vi "ExtWndAttributes.vi"(8 "EorIn":errorcluster) -> (0 "ErrOut":errorcluster)   [LabVIEW 2014]
doc: "Use this template to build a VI to use as a subVI."
panel:
  # "Output Parameters"
  # "Input Parameters"
  # "VI Description:\nThis VI is .."
  # ":: MVi Framework V1.0 ::\nAuthor:Gaoke Yang\nEmail: gaoke.yang@yahoo.com\nWeb: www.mvicontrol.com\nCopyright (C) 2015, MVI Technologies All Rights Reserved"
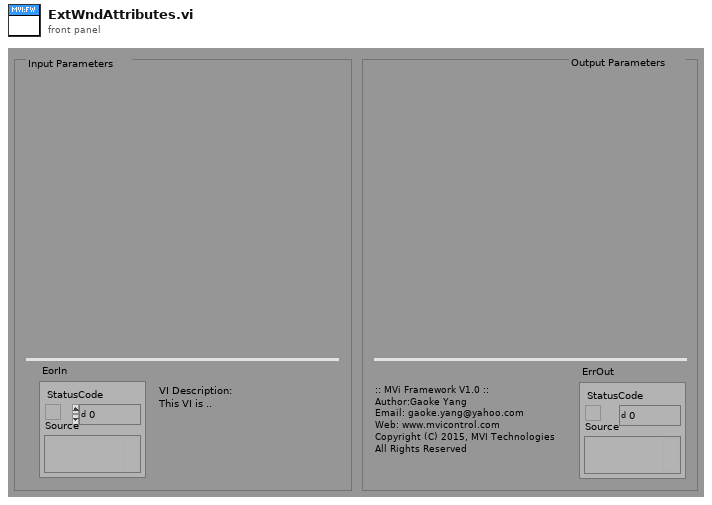
[diagram p1: front panel]
types:
  T1 = typedef "Image Type" = u32
  T2 = typedef "IMAQ Image.ctl" = refnum<image>
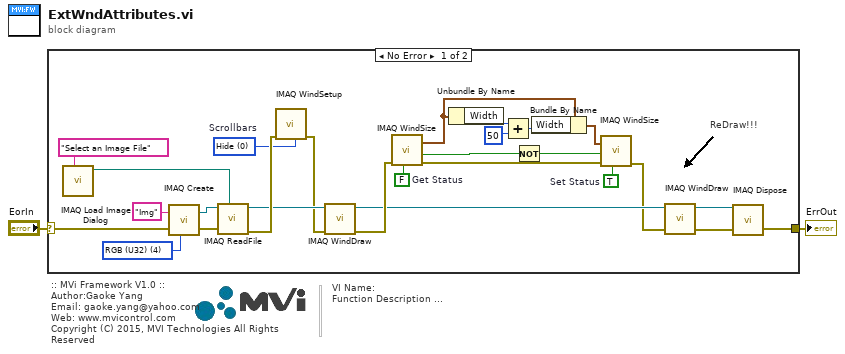
[diagram p0: block diagram]
diagram:
  # "VI Name:\nFunction Description ..."
  # ":: MVi Framework V1.0 ::\nAuthor:Gaoke Yang\nEmail: gaoke.yang@yahoo.com\nWeb: www.mvicontrol.com\nCopyright (C) 2015, MVI Technologies All Rights Reserved"
  n1 = case shown="No Error" "EorIn" {
    selector: "EorIn" -> [w4 w30]
    tunnel: [w24 w30] -> w1
    frame No Error {
      w16 = TRUE  # Set Status
      w17 = FALSE  # Get Status
      w21 = T1 4 items=["Grayscale (U8)", "Grayscale (I16)", "Grayscale (SGL)", "Complex (CSG)", "RGB (U32)", "HSL (U32)", "RGB (U64)", "Grayscale (U16)"] ("Image Type")
      w22 = 0 items=["Hide", "Show", "No change"]  # Scrollbars
      # "ReDraw!!!"
      n2 = call "IMAQ Load Image Dialog"("Prompt"="Select an Image File" ("prompt")) -> ("Path"=w23:path)  [unwired: 8 in, 2 out]
      n3 = call "IMAQ Create"("Image Name"="Img", "Image Type"=w21, "error in (no error)"=w4) -> ("New Image"=w25:T2, "error out"=w27:errorcluster)  [unwired: 2 in]
      n4 = call "IMAQ ReadFile"("File Path"=w23, "error in (no error)"=w27, "Image"=w25) -> ("error out"=w26:errorcluster, "Image Out"=w20:T2)  [unwired: 4 in, 3 out]
      n5 = call "IMAQ WindSetup"("Scrollbars (No change)"=w22, "error in (no error)"=w26) -> ("error out"=w19:errorcluster)  [unwired: 9 in]
      n6 = call "IMAQ WindDraw"("error in (no error)"=w19, "Image"=w20) -> ("error out"=w18:errorcluster, "Image Out (duplicate)"=w8:T2)  [unwired: 8 in]
      n7 = call "IMAQ WindSize"("error in (no error)"=w18, "Get/Set Status? (Set)"=w17) -> ("Has Scrollbars?"=w14:bool, "error out"=w15:errorcluster, "Width & Height out"=w10:cluster{"Width":i32, "Height":i32})  [unwired: 4 in]
      n8 = Unbundle By Name(w10) -> ("Width"=w13:i32)
      n9 = Add(x=w13, y=50) -> (x+y=w11:i32)
      n10 = Not(x=w14) -> (.not. x?=w3:bool)
      n11 = Bundle By Name(cluster=w10, "Width"=w11) -> (w9:cluster{"Width":i32, "Height":i32})
      n12 = call "IMAQ WindSize"("error in (no error)"=w15, "Scrollbars? (N)"=w3, "Get/Set Status? (Set)"=w16, "Width & Height"=w9) -> ("error out"=w6:errorcluster)  [unwired: 2 in, 2 out]
      n13 = call "IMAQ WindDraw"("error in (no error)"=w6, "Image"=w8) -> ("error out"=w5:errorcluster, "Image Out (duplicate)"=w7:T2)  [unwired: 8 in]
      n14 = call "IMAQ Dispose"("Image"=w7, "error in (no error)"=w5) -> ("error out"=w24:errorcluster)  [unwired: 4 in]
    }
    frame Error {
    }
  }
  "ErrOut" <- w1
